vi "TrajectoryCalculateOrientationTowards.vi"(5 "Starting Fraction":dbl=0.25, 6 "Init":bool, 7 "Completion Fraction":dbl=0.75, 8 "Total Trajectory Time Sec":dbl, 9 "Elapsed Traj Time Sec":dbl, 10 "Current Orientation Demand DEG":dbl, 11 "Starting Orientation  DEG":dbl) -> (1 "Rotational Velocity Rad Per Sec":dbl, 2 "Orientation Demand Deg":dbl, 3 "Orientation Demand":T1 {"SIN" format="%13.4f"; "COS" format="%13.4f"; "VALUE" format="%13.4f"})   [LabVIEW 2023]
uses:
  <vilib>/Rock Robotics/WPI/ThirdParty/JAS_Junk/TrajLib/TypeDef/ROTATION2D.ctl
  <vilib>/Rock Robotics/WPI/ThirdParty/JAS_Junk/TrajLib/Rotation2d_GetRadians.vi
  <vilib>/Rock Robotics/WPI/ThirdParty/JAS_Junk/TrajLib/Conv_Radians_Deg.vi
  <vilib>/Rock Robotics/WPI/ThirdParty/JAS_Junk/TrajLib/Rotation2d_CreateAngle.vi
  <vilib>/Rock Robotics/WPI/ThirdParty/JAS_Junk/TrajLib/Rotation2d_Plus.vi
  <vilib>/Rock Robotics/WPI/ThirdParty/JAS_Junk/TrajLib/Rotation2d_Minus.vi
  <vilib>/Rock Robotics/WPI/ThirdParty/JAS_Junk/TrajLib/Rotation2d_Times.vi
  <vilib>/Rock Robotics/WPI/ThirdParty/JAS_Junk/TrajLib/Rotation2d_RotateBy.vi
  <vilib>/Rock Robotics/WPI/ThirdParty/JAS_Junk/TrajLib/Rotation2d_UnaryMinus.vi
  <vilib>/Rock Robotics/WPI/ThirdParty/JAS_Junk/TrajLib/Rotation2d_CreateXY.vi
  <vilib>/Rock Robotics/WPI/ThirdParty/JAS_Junk/TrajLib/Util_CalcDist.vi
  <vilib>/Rock Robotics/WPI/ThirdParty/JAS_Junk/TrajLib/Trajectory_Library.lvlib
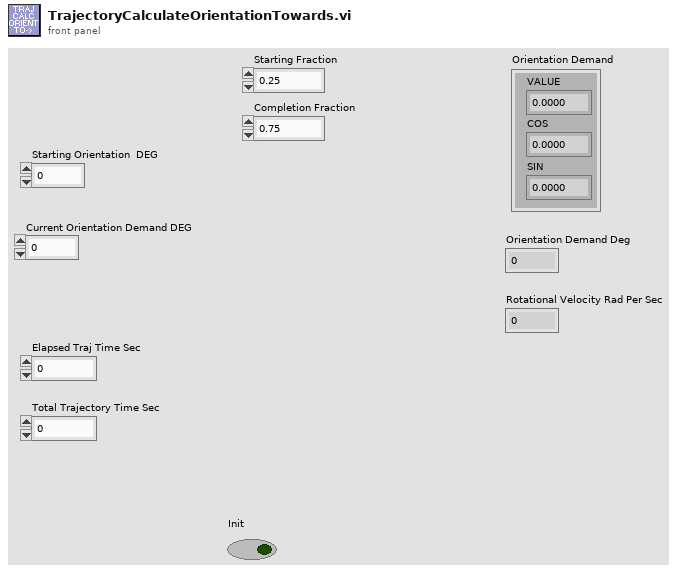
[diagram p1: front panel]
types:
  T1 = typedef "Trajectory_Library.lvlib/ROTATION2D.ctl" = cluster{"VALUE":dbl, "COS":dbl, "SIN":dbl}
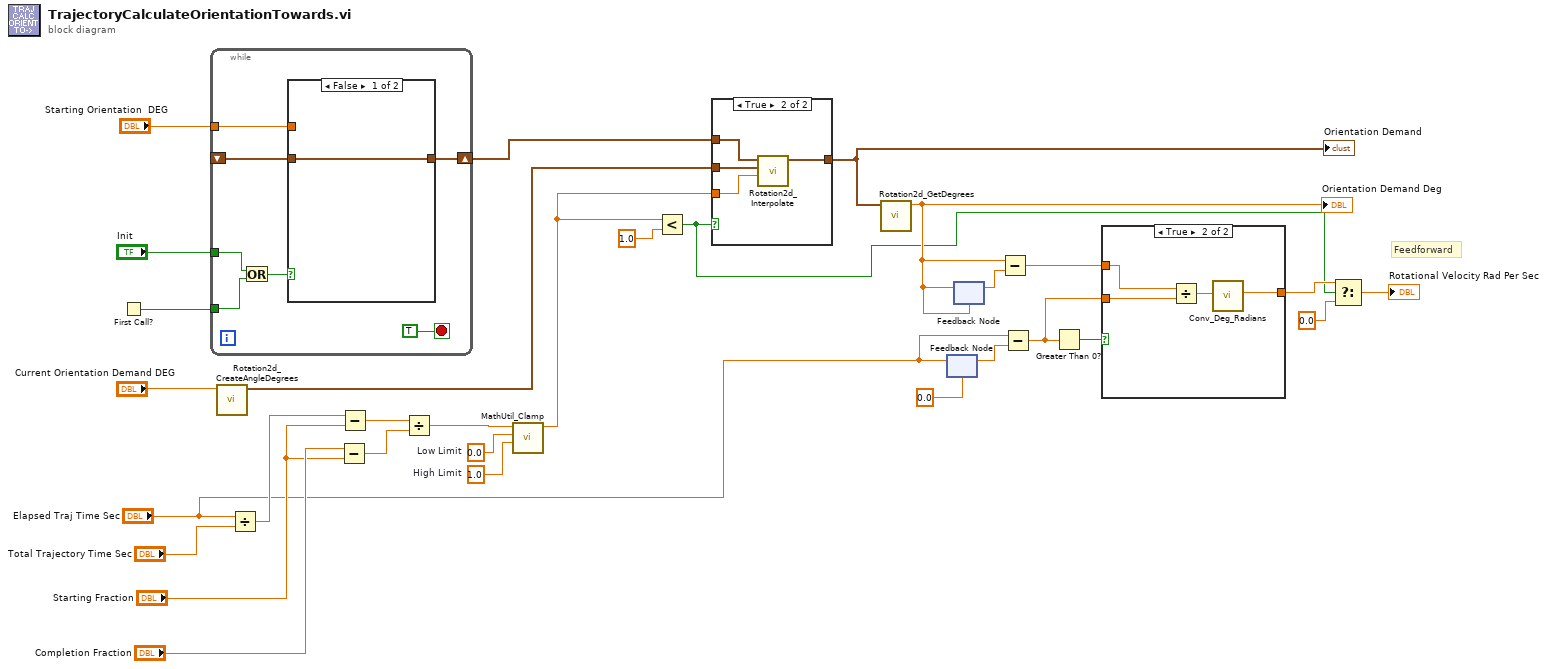
[diagram p0: block diagram]
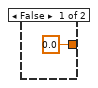
[diagram p2: hidden frame]
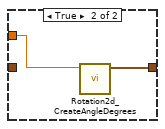
[diagram p4: hidden frame]
diagram:
  w22 = 1.0  # High Limit
  w21 = 0.0  # Low Limit
  # "Feedforward"
  n1 = First Call?() -> (First Call?: T/F=w18:bool)
  n2 = while {
    tunnel: "Init" -> [w32]
    shift-right: [w36] -> w28
    shift-left: _ -> [w35]
    tunnel: "Starting Orientation  DEG" -> [w34]
    tunnel: w18 -> [w31]
    stop <- TRUE stop-if-true
    n3 = Or(x=w32, y=w31) -> (x .or. y?=w33:bool)
    n4 = case shown="False" w33 {
      tunnel: [w38 w39] -> w36
      tunnel: w35 -> [w38 _]
      tunnel: w34 -> [_ w40]
      frame False {
      }
      frame True {
        n5 = call <vilib>:"Rotation2d_CreateAngleDegrees.vi"("Angle_Degrees"=w40) -> ("ROTATION"=w39:T1)  [unwired: 10 in]
      }
    }
  }
  n6 = call <vilib>:"Rotation2d_CreateAngleDegrees.vi"("Angle_Degrees"="Current Orientation Demand DEG") -> ("ROTATION"=w16:T1)  [unwired: 10 in]
  n7 = Divide(x="Elapsed Traj Time Sec", y="Total Trajectory Time Sec") -> (x/y=w25:dbl)
  n8 = Subtract(x="Completion Fraction", y="Starting Fraction") -> (x-y=w19:dbl)
  n9 = Subtract(x=w25, y="Starting Fraction") -> (x-y=w26:dbl)
  n10 = Divide(x=w26, y=w19) -> (x/y=w20:dbl)
  n11 = call <vilib>:"MathUtil_Clamp.vi"("High Limit"=w22, "Low Limit"=w21, "Value"=w20) -> ("Result"=w15:dbl)  [unwired: 8 in]
  n12 = Less?(x=w15, y=1.0) -> (x < y?=w3:bool)
  n13 = case shown="True" w3 {
    tunnel: w28 -> [_ w45]
    tunnel: w16 -> [w41 w44]
    tunnel: w15 -> [_ w43]
    tunnel: [w41 w42] -> w13
    frame False {
    }
    frame True {
      n14 = call <vilib>:"Rotation2d_Interpolate.vi"("T"=w43, "EncValue ROTATION"=w44, "in ROTATION"=w45) -> ("Interpolated ROTATION"=w42:T1)  [unwired: 8 in]
    }
  }
  "Orientation Demand" <- w13
  n15 = call <vilib>:"Rotation2d_GetDegrees.vi"("in ROTATION"=w13) -> ("AngleDegrees"=w12:dbl)  [unwired: 10 in]
  "Orientation Demand Deg" <- w12
  n16 = feedback #1(0.0 ("Elapsed Traj Time Sec")) -> (w8:dbl)
  n17 = feedback-in #1("Elapsed Traj Time Sec") -> ()
  n18 = feedback-in #2(w12) -> ()
  n19 = feedback #2(w12) -> (w11:dbl)
  n20 = Subtract(x=w12, y=w11) -> (x-y=w6:dbl)
  n21 = Subtract(x="Elapsed Traj Time Sec", y=w8) -> (x-y=w5:dbl)
  n22 = Greater Than 0?(x=w5) -> (x > 0?=w7:bool)
  n23 = case shown="True" w7 {
    tunnel: w6 -> [_ w50]
    tunnel: w5 -> [_ w49]
    tunnel: [0.0 ("Radians") w47] -> w4
    frame False {
    }
    frame True {
      n24 = Divide(x=w50, y=w49) -> (x/y=w48:dbl)
      n25 = call <vilib>:"Conv_Deg_Radians.vi"("Degress"=w48) -> ("Radians"=w47:dbl)  [unwired: 10 in]
    }
  }
  n26 = Select(t=w4, s=w3, f=0.0) -> (s? t:f=→"Rotational Velocity Rad Per Sec":dbl)
